vi "PCI1220U初始化.vi"() -> (4 "DeviceHandle":u32, 6 "上下拖动伺服":u32, 8 "输入轴伺服":u32, 10 "DeviceNum List":u32[](array[numeric]), 15 "DevAxesCount":u32)   [LabVIEW 2013]
panel:
  out "Error Output 2":errorcluster caption="Error Output"
  out "Error Output":errorcluster
  out "ReturnValue 8":u32
  out "ReturnValue 7":u32
  out "ReturnValue 6":u32
  out "ReturnValue 5":u32
  out "ReturnValue 4":u32
  out "ReturnValue 3":u32
  out "ReturnValue 2":u32
  out "ReturnValue":u32
  out "Device Type 2":u16(ring) items=["PCI-1220 (M0)"]
  out "AxisOpened":bool
  in  "Device Type":u16(ring) items=["PCI-1220 (M0)"]
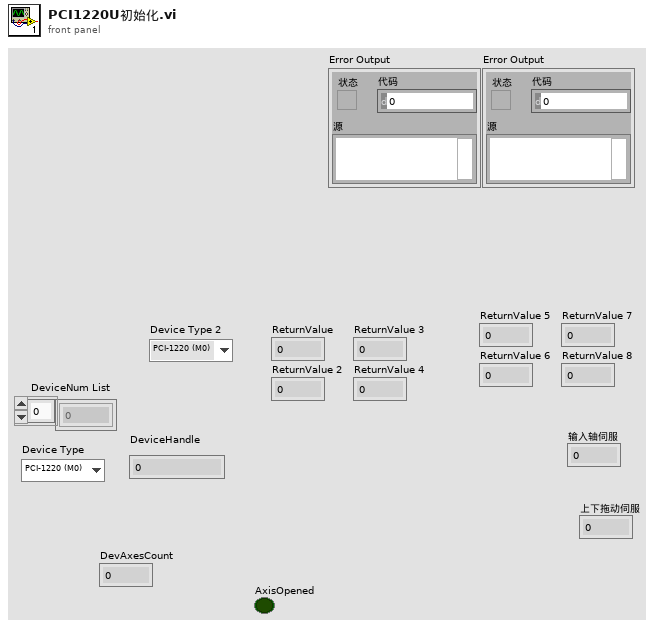
[diagram p1: front panel]
types:
  T1 = cluster{"DeviceNum":u32, "U*8 Array":cluster{"U*8 Array[0]":u8, "U*8 Array[1]":u8, "U*8 Array[2]":u8, "U*8 Array[3]":u8, "U*8 Array[4]":u8, "U*8 Array[5]":u8, "U*8 Array[6]":u8, "U*8 Array[7]":u8, "U*8 Array[8]":u8, "U*8 Array[9]":u8, "U*8 Array[10]":u8, "U*8 Array[11]":u8, "U*8 Array[12]":u8, "U*8 Array[13]":u8, "U*8 Array[14]":u8, "U*8 Array[15]":u8, "U*8 Array[16]":u8, "U*8 Array[17]":u8, "U*8 Array[18]":u8, "U*8 Array[19]":u8, "U*8 Array[20]":u8, "U*8 Array[21]":u8, "U*8 Array[22]":u8, "U*8 Array[23]":u8, "U*8 Array[24]":u8, "U*8 Array[25]":u8, "U*8 Array[26]":u8, "U*8 Array[27]":u8, "U*8 Array[28]":u8, "U*8 Array[29]":u8, "U*8 Array[30]":u8, "U*8 Array[31]":u8, "U*8 Array[32]":u8, "U*8 Array[33]":u8, "U*8 Array[34]":u8, "U*8 Array[35]":u8, "U*8 Array[36]":u8, "U*8 Array[37]":u8, "U*8 Array[38]":u8, "U*8 Array[39]":u8, "U*8 Array[40]":u8, "U*8 Array[41]":u8, "U*8 Array[42]":u8, "U*8 Array[43]":u8, "U*8 Array[44]":u8, "U*8 Array[45]":u8, "U*8 Array[46]":u8, "U*8 Array[47]":u8, "U*8 Array[48]":u8, "U*8 Array[49]":u8}, "NumOfSubDevice":i16}[]
  T2 = cluster{"U*8 Array[0]":u8, "U*8 Array[1]":u8, "U*8 Array[2]":u8, "U*8 Array[3]":u8, "U*8 Array[4]":u8, "U*8 Array[5]":u8, "U*8 Array[6]":u8, "U*8 Array[7]":u8, "U*8 Array[8]":u8, "U*8 Array[9]":u8, "U*8 Array[10]":u8, "U*8 Array[11]":u8, "U*8 Array[12]":u8, "U*8 Array[13]":u8, "U*8 Array[14]":u8, "U*8 Array[15]":u8, "U*8 Array[16]":u8, "U*8 Array[17]":u8, "U*8 Array[18]":u8, "U*8 Array[19]":u8, "U*8 Array[20]":u8, "U*8 Array[21]":u8, "U*8 Array[22]":u8, "U*8 Array[23]":u8, "U*8 Array[24]":u8, "U*8 Array[25]":u8, "U*8 Array[26]":u8, "U*8 Array[27]":u8, "U*8 Array[28]":u8, "U*8 Array[29]":u8, "U*8 Array[30]":u8, "U*8 Array[31]":u8, "U*8 Array[32]":u8, "U*8 Array[33]":u8, "U*8 Array[34]":u8, "U*8 Array[35]":u8, "U*8 Array[36]":u8, "U*8 Array[37]":u8, "U*8 Array[38]":u8, "U*8 Array[39]":u8, "U*8 Array[40]":u8, "U*8 Array[41]":u8, "U*8 Array[42]":u8, "U*8 Array[43]":u8, "U*8 Array[44]":u8, "U*8 Array[45]":u8, "U*8 Array[46]":u8, "U*8 Array[47]":u8, "U*8 Array[48]":u8, "U*8 Array[49]":u8}
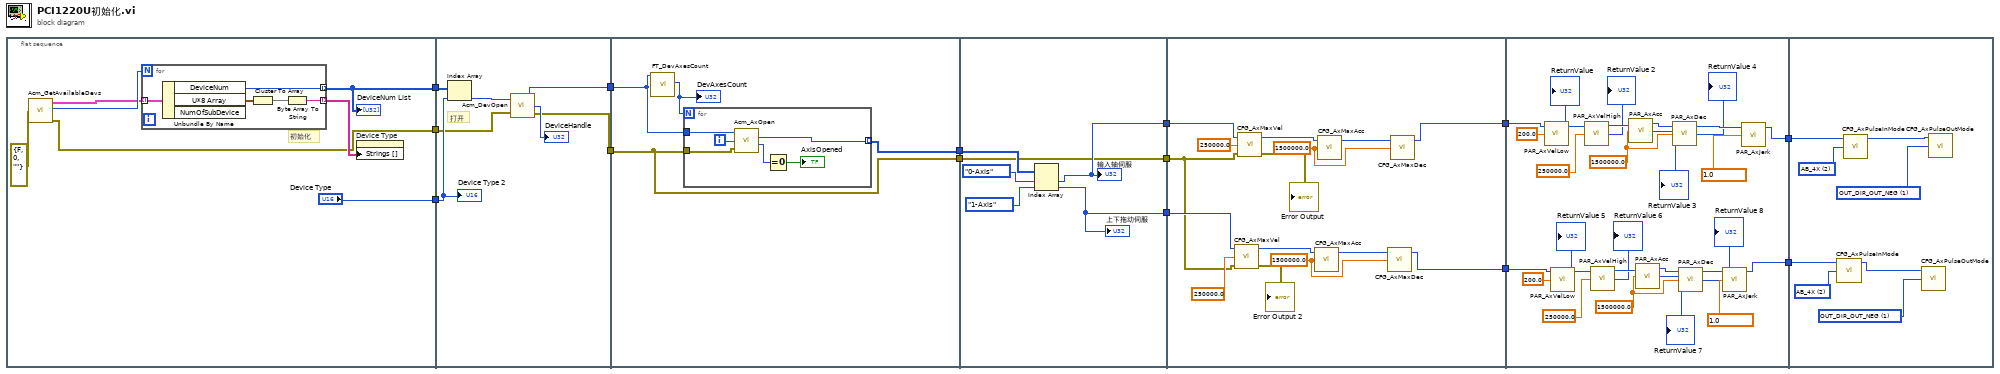
[diagram p0: block diagram]
diagram:
  n1 = flat-sequence {
    tunnel: [w18] -> w14
    tunnel: ["Device Type"] -> w13
    tunnel: [w15] -> w4
    tunnel: w14 -> [w33]
    tunnel: w13 -> [w29]
    tunnel: [w31] -> w12
    tunnel: w4 -> [w28]
    tunnel: [w27] -> w3
    tunnel: w12 -> [w36]
    tunnel: [w35] -> w11
    tunnel: w3 -> [w34]
    tunnel: [w34] -> w1
    tunnel: w11 -> [w49]
    tunnel: [w47] -> w10
    tunnel: [w45] -> w8
    tunnel: [w44] -> w2
    tunnel: w1 -> [w44]
    tunnel: w10 -> [w60]
    tunnel: [w59] -> w9
    tunnel: w8 -> [w54]
    tunnel: [w53] -> w7
    tunnel: w2 -> [w52]
    tunnel: w9 -> [w92]
    tunnel: w7 -> [w67]
    tunnel: [w66] -> w6
    tunnel: [w65] -> w5
    tunnel: w6 -> [w100]
    tunnel: w5 -> [w97]
    frame #0 {
      # "初始化"
      n2 = call <userlib>:"Acm_GetAvailableDevs.vi"("Error Input(No Error)"=errorcluster {"status"=FALSE, "code"=0, "source"=""}) -> ("Error Output"=w15:errorcluster, "OutEntries"=w21:u32, "DeviceList"=w20:T1)  [unwired: 1 out]
      n3 = for {
        N: w21 -> [_]
        tunnel: w20 -> [w26] mode=indexing
        tunnel: [w23] -> w18 mode=indexing
        tunnel: [w22] -> w19 mode=indexing
        n4 = Unbundle By Name(w26) -> ("DeviceNum"=w23:u32, "U*8 Array"=w25:T2)  [unwired: 1 out]
        n5 = Cluster To Array(cluster=w25) -> (array=w24:u8[])
        n6 = Byte Array To String(unsigned byte array=w24) -> (string=w22:string)
      }
      "DeviceNum List" <- w18
      n7 = property on="Device Type" class="Ring (严格)"("Strings []"=w19) -> ()  [unwired: 2 in, 2 out]
    }
    frame #1 {
      # "打开"
      n8 = Index Array(array=w33, index=w29) -> (element=w32:u32)
      n9 = call <userlib>:"Acm_DevOpen.vi"("Error Input(No Error)"=w28, "DeviceNumber"=w32) -> ("Error Output"=w27:errorcluster, "ReturnValue"=→"DeviceHandle":u32, "DeviceHandle"=w31:u32)
      "Device Type 2" <- w29
    }
    frame #2 {
      n10 = call <userlib>:"FT_DevAxesCount.vi"("Handle"=w36) -> ("DevAxesCount"=w37:u32)  [unwired: 1 in, 6 out]
      "DevAxesCount" <- w37
      n11 = for {
        N: w37 -> [_]
        tunnel: w36 -> [w43]
        tunnel: [w39] -> w35 mode=indexing
        tunnel: w34 -> [w38]
        i -> [w42]
        n12 = call <userlib>:"Acm_AxOpen.vi"("Error Input(No Error)"=w38, "PhyAxis"=w42, "DeviceHandle"=w43) -> ("ReturnValue"=w41:u32, "AxisHandle"=w39:u32)  [unwired: 2 out]
        n13 = Equal To 0?(x=w41) -> (x = 0?=→"AxisOpened":bool)
      }
    }
    frame #3 {
      n14 = Index Array(array=w49, index #1=enum32{"0-Axis", "1-Axis", "2-Axis", "3-Axis"}."0-Axis" ("Operate Axis"), index #2=enum32{"0-Axis", "1-Axis", "2-Axis", "3-Axis"}."1-Axis" ("Operate Axis")) -> (element #1=w47:u32, element #2=w45:u32)
      "输入轴伺服" <- w47
      "上下拖动伺服" <- w45
    }
    frame #4 {
      w58 = 1500000.0 ("CFG_AxMaxAcc")
      w64 = 1500000.0 ("CFG_AxMaxAcc")
      n15 = call <userlib>:"CFG_AxMaxVel.vi"("Error Input(No Error)"=w52, "CFG_AxMaxVel"=250000.0, "Handle"=w54) -> ("Error Output"=→"Error Output 2":errorcluster, "Handle 2"=w56:u32)  [unwired: 1 out]
      n16 = call <userlib>:"CFG_AxMaxVel.vi"("Error Input(No Error)"=w52, "CFG_AxMaxVel"=250000.0, "Handle"=w60) -> ("Error Output"=→"Error Output":errorcluster, "Handle 2"=w62:u32)  [unwired: 1 out]
      n17 = call <userlib>:"CFG_AxMaxAcc.vi"("CFG_AxMaxAcc"=w58, "Handle"=w56) -> ("Handle 2"=w57:u32)  [unwired: 1 in, 2 out]
      n18 = call <userlib>:"CFG_AxMaxAcc.vi"("CFG_AxMaxAcc"=w64, "Handle"=w62) -> ("Handle 2"=w63:u32)  [unwired: 1 in, 2 out]
      n19 = call <userlib>:"CFG_AxMaxDec.vi"("CFG_AxMaxDec"=w58, "Handle"=w57) -> ("Handle 2"=w53:u32)  [unwired: 1 in, 2 out]
      n20 = call <userlib>:"CFG_AxMaxDec.vi"("CFG_AxMaxDec"=w64, "Handle"=w63) -> ("Handle 2"=w59:u32)  [unwired: 1 in, 2 out]
    }
    frame #5 {
      w72 = 1.0 items=["T-curve", "S-curve"] ("PAR_AxJerk")
      w73 = 1500000.0 ("PAR_AxAcc")
      w84 = 1.0 items=["T-curve", "S-curve"] ("PAR_AxJerk")
      w85 = 1500000.0 ("PAR_AxAcc")
      n21 = call <userlib>:"PAR_AxVelLow.vi"("PAR_AxVelLow"=200.0, "Handle"=w92) -> ("ReturnValue"=→"ReturnValue":u32, "Handle 2"=w91:u32)  [unwired: 1 in, 1 out]
      n22 = call <userlib>:"PAR_AxVelLow.vi"("PAR_AxVelLow"=200.0, "Handle"=w67) -> ("ReturnValue"=→"ReturnValue 5":u32, "Handle 2"=w79:u32)  [unwired: 1 in, 1 out]
      n23 = call <userlib>:"PAR_AxVelHigh.vi"("PAR_AxVelHigh"=250000.0, "Handle"=w91) -> ("ReturnValue"=→"ReturnValue 2":u32, "Handle 2"=w90:u32)  [unwired: 1 in, 1 out]
      n24 = call <userlib>:"PAR_AxVelHigh.vi"("PAR_AxVelHigh"=250000.0, "Handle"=w79) -> ("ReturnValue"=→"ReturnValue 6":u32, "Handle 2"=w78:u32)  [unwired: 1 in, 1 out]
      n25 = call <userlib>:"PAR_AxAcc.vi"("PAR_AxAcc"=w85, "Handle"=w90) -> ("ReturnValue"=→"ReturnValue 3":u32, "Handle 2"=w89:u32)  [unwired: 1 in, 1 out]
      n26 = call <userlib>:"PAR_AxAcc.vi"("PAR_AxAcc"=w73, "Handle"=w78) -> ("ReturnValue"=→"ReturnValue 7":u32, "Handle 2"=w77:u32)  [unwired: 1 in, 1 out]
      n27 = call <userlib>:"PAR_AxDec.vi"("PAR_AxDec"=w85, "Handle"=w89) -> ("ReturnValue"=→"ReturnValue 4":u32, "Handle 2"=w88:u32)  [unwired: 1 in, 1 out]
      n28 = call <userlib>:"PAR_AxDec.vi"("PAR_AxDec"=w73, "Handle"=w77) -> ("ReturnValue"=→"ReturnValue 8":u32, "Handle 2"=w76:u32)  [unwired: 1 in, 1 out]
      n29 = call <userlib>:"PAR_AxJerk.vi"("PAR_AxJerk"=w72, "Handle"=w76) -> ("Handle 2"=w65:u32)  [unwired: 1 in, 2 out]
      n30 = call <userlib>:"PAR_AxJerk.vi"("PAR_AxJerk"=w84, "Handle"=w88) -> ("Handle 2"=w66:u32)  [unwired: 1 in, 2 out]
    }
    frame #6 {
      w93 = u32 1 items=["OUT_DIR", "OUT_DIR_OUT_NEG", "OUT_DIR_DIR_NEG", "OUT_DIR_ALL_NEG", "O_CW_CCW", "CW_CCW_ALL_NEG", "AB_PHASE", "BA_PHASE", "CW_CCW_OUT_NEG", "CW_CCW_DIR_NEG"] ("CFG_AxPulseOutMode")
      w94 = u32 1 items=["OUT_DIR", "OUT_DIR_OUT_NEG", "OUT_DIR_DIR_NEG", "OUT_DIR_ALL_NEG", "O_CW_CCW", "CW_CCW_ALL_NEG", "AB_PHASE", "BA_PHASE", "CW_CCW_OUT_NEG", "CW_CCW_DIR_NEG"] ("CFG_AxPulseOutMode")
      w95 = u32 2 items=["AB_1X", "AB_2X", "AB_4X", "I_CW_CCW"] ("CFG_AxPulseInMode")
      w98 = u32 2 items=["AB_1X", "AB_2X", "AB_4X", "I_CW_CCW"] ("CFG_AxPulseInMode")
      n31 = call <userlib>:"CFG_AxPulseInMode.vi"("CFG_AxPulseInMode"=w95, "Handle"=w97) -> ("Handle 2"=w96:u32)  [unwired: 1 in, 2 out]
      n32 = call <userlib>:"CFG_AxPulseInMode.vi"("CFG_AxPulseInMode"=w98, "Handle"=w100) -> ("Handle 2"=w99:u32)  [unwired: 1 in, 2 out]
      n33 = call <userlib>:"CFG_AxPulseOutMode.vi"("CFG_AxPulseOutMode"=w93, "Handle"=w96) -> ()  [unwired: 1 in, 3 out]
      n34 = call <userlib>:"CFG_AxPulseOutMode.vi"("CFG_AxPulseOutMode"=w94, "Handle"=w99) -> ()  [unwired: 1 in, 3 out]
    }
  }
